vi "Assert Content is Correct.vi"(5 "Assert Only? (F)":bool, 6 "error code (1)":i32=1, 7 "Label":string="Content is correct", 8 "Error In":errorcluster, 10 "Expected":string, 11 "Token":refnum<class "Abstract.lvclass">) -> (0 "Error Out":errorcluster)   [LabVIEW 2018, in "Tests.lvlib"]
uses:
  Tests.lvlib
  src/Mustache/Public/Tokens/Public/Abstract/Abstract.lvclass
  src/Mustache/Public/Tokens/Public/Text/Text.lvclass
  <vilib>/addons/_JKI Toolkits/Caraya/classes/Assert/Assert.lvclass
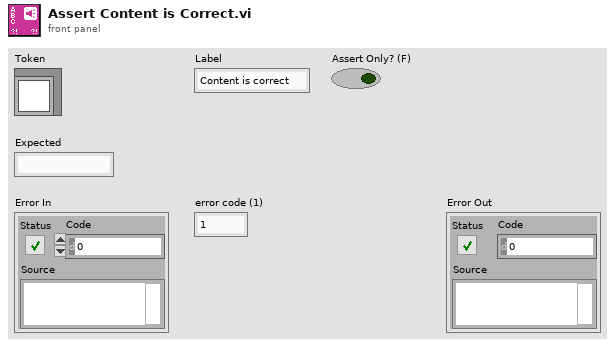
[diagram p1: front panel]
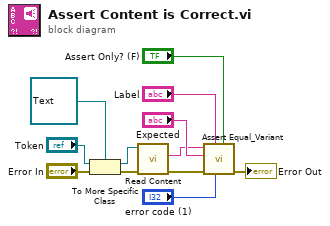
[diagram p0: block diagram]
diagram:
  n1 = To More Specific Class(target class=refnum<class "Text.lvclass"> refnum ("Mustache.lvlib:Tokens.lvlib:Text.lvclass"), reference="Token", error in="Error In") -> (specific class reference=w1:refnum<class "Text.lvclass">, error out=w6:errorcluster)
  n2 = call "Read Content.vi"("Error In"=w6, "Text In"=w1) -> ("Error Out"=w7:errorcluster, "Content"=w8:string)  [unwired: 7 in, 1 out]
  n3 = call <vilib>:"Assert Equal_Variant.vi"("Assert Only? (F)"="Assert Only? (F)", "error code (1)"="error code (1)", "Label"="Label", "error in (no error)"=w7, "Y"="Expected", "X"=w8) -> ("error out"=→"Error Out":errorcluster)  [unwired: 5 in]
